vi "zahvat_cont.vi"   [LabVIEW 2017]
uses:
  <vilib>/myRIO/Instrument Drivers/Onboard IO/DIO/typedefs/DIO Reference.ctl
  <vilib>/myRIO/Common/Instrument Driver Framework/Utilities/typedefs/myRIO Generic Hardware Reference.ctl
  <vilib>/myRIO/Common/Instrument Driver Framework/Utilities/typedefs/Hardware Version Enum.ctl
  <vilib>/myRIO/Common/Instrument Driver Framework/Utilities/typedefs/myRIO v1.0 Reference.ctl
  <vilib>/myRIO/Common/Instrument Driver Framework/Utilities/typedefs/Generic FPGA Reference.ctl
  <vilib>/myRIO/Common/Instrument Driver Framework/myRIO v1.0/DIO/typedefs/DIO Channels List.ctl
  <vilib>/myRIO/Common/Instrument Driver Framework/myRIO v1.0/DIO/typedefs/DIO Channels Enum.ctl
  <vilib>/userdefined/High Color/nirio_resource_hc.ctl
  <vilib>/myRIO/Instrument Drivers/Onboard IO/PWM/typedefs/PWM Reference.ctl
  <vilib>/myRIO/Common/Instrument Driver Framework/myRIO v1.0/PWM/typedefs/PWM Channels Enum.ctl
  <vilib>/myRIO/Instrument Drivers/Onboard IO/PWM/typedefs/PWM Configuration.ctl
  <vilib>/myRIO/Common/Instrument Driver Framework/Utilities/vis/Is FPGA Ref Available.vi
  <vilib>/myRIO/Common/Instrument Driver Framework/myRIO v1.0/DIO/vis/myRIO v1.1 Open DIO.vi
  <vilib>/myRIO/Instrument Drivers/Onboard IO/DIO/vis/Write.vi
  <vilib>/myRIO/Common/Instrument Driver Framework/myRIO v1.0/PWM/vis/myRIO v1.1 Open PWM.vi
  <vilib>/myRIO/Instrument Drivers/Onboard IO/PWM/vis/Set Duty Cycle and Frequency.vi
  <vilib>/myRIO/Common/Instrument Driver Framework/Utilities/vis/Validate Channels.vi
  <vilib>/myRIO/Common/Instrument Driver Framework/myRIO v1.0/DIO/vis/myRIO v1.0 Reserve DIO.vi
  <vilib>/myRIO/Common/Instrument Driver Framework/myRIO v1.0/PWM/vis/myRIO v1.0 Reserve PWM.vi
  <vilib>/myRIO/Common/Instrument Driver Framework/myRIO v1.0/Resource Manager/vis/myRIO v1.0 Reserve Channel List.vi
  <vilib>/myRIO/Common/Instrument Driver Framework/myRIO v1.0/DIO/vis/myRIO v1.0 Build MUX Configuration DIO.vi
  <vilib>/myRIO/Common/Instrument Driver Framework/myRIO v1.0/PWM/vis/myRIO v1.0 Build MUX Configuration PWM.vi
  <vilib>/myRIO/Common/Instrument Driver Framework/myRIO v1.0/Resource Manager/vis/myRIO v1.0 Reserve Channel.vi
  <vilib>/myRIO/Common/Instrument Driver Framework/myRIO v1.0/Resource Manager/vis/myRIO v1.0 Unreserve Channel.vi
  <vilib>/myRIO/Common/Instrument Driver Framework/myRIO v1.0/Resource Manager/vis/myRIO v1.0 Create Configuration List.vi
  <vilib>/myRIO/Common/Instrument Driver Framework/myRIO v1.0/Resource Manager/vis/myRIO v1.0 Build Mutex Name.vi
  <vilib>/Utility/VariantDataType/GetNumericInfo.vi
  <vilib>/Utility/error.llb/Error Cluster From Error Code.vi
  <vilib>/myRIO/Common/Instrument Driver Framework/myRIO v1.0/myRIO v1.1 Open.vi
  <vilib>/myRIO/Common/Instrument Driver Framework/Utilities/vis/IO Manager.vi
  <vilib>/myRIO/Common/Instrument Driver Framework/Utilities/vis/Configuration Manager.vi
  <vilib>/myRIO/Common/Instrument Driver Framework/myRIO v1.0/Resource Manager/vis/myRIO v1.0 Configure IO.vi
  <vilib>/myRIO/Common/Instrument Driver Framework/myRIO v1.0/myRIO v1.0 Close.vi
  <vilib>/myRIO/Common/Instrument Driver Framework/myRIO v1.0/DIO/vis/myRIO v1.0 Write DIO.vi
  <vilib>/myRIO/Common/Instrument Driver Framework/myRIO v1.0/PWM/vis/myRIO v1.0 Write PWM.vi
  <vilib>/myRIO/Express VI/Onboard Devices/LED/LED Express VI.xnode
  <vilib>/myRIO/Instrument Drivers/Onboard IO/DIO/vis/myRIO DIO Open.xnode
  <vilib>/myRIO/Express VI/Onboard IO/PWM/PWM Express VI.xnode
  <vilib>/myRIO/Instrument Drivers/Onboard IO/PWM/vis/myRIO PWM Open.xnode
  <vilib>/myRIO/Instrument Drivers/Onboard IO/PWM/PWM.lvlib
  <vilib>/myRIO/Instrument Drivers/Onboard IO/DIO/DIO.lvlib
types:
  T1 = typedef "DIO.lvlib/DIO Reference.ctl" = cluster{"myRIO Reference":T2, "DIO Channels List":T6}
  T2 = typedef "myRIO Generic Hardware Reference.ctl" = cluster{"myRIO Model":T3, "myRIO Hardware Reference":T4}
  T3 = typedef "Hardware Version Enum.ctl" = enum16{"Unknown", "myRIO-1900", "myRIO-1950", "roboRIO", "NI ELVIS RIO CM"}
  T4 = typedef "myRIO v1.0 Reference.ctl" = cluster{"Generic FPGA Reference":T5, "Allow multiple opens":bool}
  T5 = typedef "Generic FPGA Reference.ctl" = refnum<k20>
  T6 = typedef "DIO Channels List.ctl" = T7[]
  T7 = typedef "DIO Channels Enum.ctl" = enum16{"Not Connected", "C/DIO0", "C/DIO1", "C/DIO2", "C/DIO3", "C/DIO4", "C/DIO5", "C/DIO6", "C/DIO7", "A/DIO0", "A/DIO1", "A/DIO2", "A/DIO3", "A/DIO4", "A/DIO5", "A/DIO6", "A/DIO7", "A/DIO8", "A/DIO9", "A/DIO10", "A/DIO11", "A/DIO12", "A/DIO13", "A/DIO14", "A/DIO15", "B/DIO0", "B/DIO1", "B/DIO2", "B/DIO3", "B/DIO4", "B/DIO5", "B/DIO6", "B/DIO7", "B/DIO8", "B/DIO9", "B/DIO10", "B/DIO11", "B/DIO12", "B/DIO13", "B/DIO14", "B/DIO15", "LED0", "LED1", "LED2", "LED3", "Button0", "DIO/DIO0", "DIO/DIO1", "DIO/DIO2", "DIO/DIO3", "DIO/DIO4", "DIO/DIO5", "DIO/DIO6", "DIO/DIO7", "DIO/DIO8", "DIO/DIO9", "SPI/CS0", "SPI/CS1", "SPI/CS2", "SPI/CS3", "LED RADIO (Green)", "LED RADIO (Red)", "LED COMM (Green)", "LED COMM (Red)", "LED MODE (Green)", "LED MODE (Red)"}
  T8 = typedef "nirio_resource_hc.ctl" = tag
  T9 = typedef "PWM.lvlib/PWM Reference.ctl" = cluster{"myRIO Reference":T2, "PWM Channels Enum":T10, "PWM Configuration":T11}
  T10 = typedef "PWM Channels Enum.ctl" = enum16{"Not Connected", "C/PWM0", "C/PWM1", "A/PWM0", "A/PWM1", "A/PWM2", "B/PWM0", "B/PWM1", "B/PWM2", "PWM/PWM0", "PWM/PWM1", "PWM/PWM2", "PWM/PWM3", "PWM/PWM4", "PWM/PWM5", "PWM/PWM6", "PWM/PWM7", "PWM/PWM8", "PWM/PWM9"}
  T11 = typedef "PWM.lvlib/PWM Configuration.ctl" = cluster{"Frequency":dbl, "Duty Cycle":dbl}
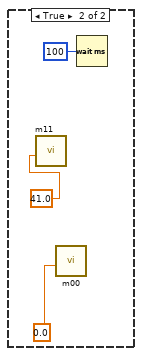
[diagram p3: hidden frame]
diagram:
  n1 = flat-sequence {
    frame #0 {
      n2 = Wait (ms)(milliseconds to wait=u32 1000) -> ()  [unwired: 1 out]
    }
    frame #1 {
      n3 = while {
        stop <- w3 stop-if-true
        n4 = call "ir2.vi"("Koffset [cm]"=0.0, "Kscale [cm-V]"=27.5) -> ("см"=w5:dbl)  [unwired: 8 in, 1 out]
        n5 = Less Or Equal?(x=w5, y=40.0) -> (x <= y?=w2:bool)
        n6 = case shown="True" w2 {
          frame False {
          }
          frame True {
            n7 = Wait (ms)(milliseconds to wait=u32 3000) -> ()  [unwired: 1 out]
          }
        }
        n8 = Not(x=w2) -> (.not. x?=w3:bool)
      }
    }
    frame #2 {
      n9 = flat-sequence {
        frame #0 {
          n10 = call "m11.vi"("position"=49.0) -> ()  [unwired: 10 in, 1 out]
          n11 = call "m00.vi"("position"=38.0) -> ()  [unwired: 10 in, 1 out]
          n12 = Wait (ms)(milliseconds to wait=u32 1650) -> ()  [unwired: 1 out]
        }
        frame #1 {
          n13 = call "m11.vi"("position"=0.0) -> ()  [unwired: 10 in, 1 out]
          n14 = call "m00.vi"("position"=0.0) -> ()  [unwired: 10 in, 1 out]
          n15 = Wait (ms)(milliseconds to wait=u32 1000) -> ()  [unwired: 1 out]
        }
        frame #2 {
          n16 = call "m00.vi"("position"=40.0) -> ()  [unwired: 10 in, 1 out]
          n17 = call "m11.vi"("position"=48.0) -> ()  [unwired: 10 in, 1 out]
          n18 = Wait (ms)(milliseconds to wait=u32 2950) -> ()  [unwired: 1 out]
        }
        frame #3 {
          w18 = TRUE ("LED0")
          n19 = call "m11.vi"("position"=0.0) -> ()  [unwired: 10 in, 1 out]
          n20 = xnode "LED"("LED0"=w18, "LED1"=w18, "LED2"=w18, "LED3"=w18) -> ()  [unwired: 1 in, 1 out]
          n21 = call "m00.vi"("position"=0.0) -> ()  [unwired: 10 in, 1 out]
          n22 = Wait (ms)(milliseconds to wait=u32 10000) -> ()  [unwired: 1 out]
        }
        frame #4 {
          w60 = FALSE ("LED0")
          n23 = xnode "LED 2"("LED0"=w60, "LED1"=w60, "LED2"=w60, "LED3"=w60) -> ()  [unwired: 1 in, 1 out]
        }
        frame #5 {
          n24 = call "line_sensor.vi"() -> ("line_true"=w99:bool)  [unwired: 10 in, 1 out]
          n25 = case shown="False" w99 {
            frame False {
              n26 = call "m11.vi"("position"=0.0) -> ()  [unwired: 10 in, 1 out]
              n27 = call "m00.vi"("position"=41.0) -> ()  [unwired: 10 in, 1 out]
              n28 = Wait (ms)(milliseconds to wait=u32 100) -> ()  [unwired: 1 out]
            }
            frame True {
              n29 = call "m11.vi"("position"=41.0) -> ()  [unwired: 10 in, 1 out]
              n30 = call "m00.vi"("position"=0.0) -> ()  [unwired: 10 in, 1 out]
              n31 = Wait (ms)(milliseconds to wait=u32 100) -> ()  [unwired: 1 out]
            }
          }
        }
        frame #6 {
          n32 = call "m11.vi"("position"=0.0) -> ()  [unwired: 10 in, 1 out]
          n33 = call "m00.vi"("position"=0.0) -> ()  [unwired: 10 in, 1 out]
        }
        frame #7 {
        }
        frame #8 {
          n34 = call "m11.vi"("position"=0.0) -> ()  [unwired: 10 in, 1 out]
          n35 = call "m00.vi"("position"=0.0) -> ()  [unwired: 10 in, 1 out]
          n36 = Wait (ms)(milliseconds to wait=u32 1000) -> ()  [unwired: 1 out]
        }
        frame #9 {
        }
      }
    }
    frame #3 {
      n37 = Wait (ms)(milliseconds to wait=u32 1000) -> ()  [unwired: 1 out]
    }
    frame #4 {
      n38 = while {
        stop <- w112 stop-if-true
        # "2,3"
        n39 = flat-sequence {
          tunnel: [w120] -> w117
          tunnel: [w133] -> w118
          tunnel: [w140] -> w116
          tunnel: [w146] -> w113
          frame #0 {
            n40 = while {
              tunnel: [w124] -> w120
              stop <- w126 stop-if-true
              # "37,5"
              # "37"
              n41 = call "m00.vi"("position"=40.0) -> ()  [unwired: 10 in, 1 out]
              n42 = call "m11.vi"("position"=0.0) -> ()  [unwired: 10 in, 1 out]
              n43 = call "line_sensor.vi"() -> ("line_true"=w126:bool)  [unwired: 10 in, 1 out]
              n44 = call "ir.vi"("Koffset [cm]"=0.0, "Kscale [cm-V]"=27.5) -> ("см"=w125:dbl)  [unwired: 8 in, 1 out]
              n45 = Less Or Equal?(x=w125, y=15.0) -> (x <= y?=w124:bool)
            }
            n46 = Wait (ms)(milliseconds to wait=u32 10) -> ()  [unwired: 1 out]
          }
          frame #1 {
            n47 = Wait (ms)(milliseconds to wait=u32 10) -> ()  [unwired: 1 out]
            n48 = call "m00.vi"("position"=0.0) -> ()  [unwired: 10 in, 1 out]
            n49 = call "ir.vi"("Koffset [cm]"=0.0, "Kscale [cm-V]"=27.5) -> ("см"=w134:dbl)  [unwired: 8 in, 1 out]
            n50 = call "m11.vi"("position"=0.0) -> ()  [unwired: 10 in, 1 out]
            n51 = Less Or Equal?(x=w134, y=15.0) -> (x <= y?=w133:bool)
          }
          frame #2 {
            # "37,5"
            # "41"
            n52 = call "m00.vi"("position"=0.0) -> ()  [unwired: 10 in, 1 out]
            n53 = call "m11.vi"("position"=41.0) -> ()  [unwired: 10 in, 1 out]
            n54 = call "ir.vi"("Koffset [cm]"=0.0, "Kscale [cm-V]"=27.5) -> ("см"=w141:dbl)  [unwired: 8 in, 1 out]
            n55 = Less Or Equal?(x=w141, y=15.0) -> (x <= y?=w140:bool)
            n56 = Wait (ms)(milliseconds to wait=u32 30) -> ()  [unwired: 1 out]
          }
          frame #3 {
            n57 = call "ir.vi"("Koffset [cm]"=0.0, "Kscale [cm-V]"=27.5) -> ("см"=w150:dbl)  [unwired: 8 in, 1 out]
            n58 = Less Or Equal?(x=w150, y=15.0) -> (x <= y?=w146:bool)
            n59 = call "m00.vi"("position"=0.0) -> ()  [unwired: 10 in, 1 out]
            n60 = call "m11.vi"("position"=0.0) -> ()  [unwired: 10 in, 1 out]
            n61 = Wait (ms)(milliseconds to wait=u32 10) -> ()  [unwired: 1 out]
          }
        }
        n62 = Or(x=w118, y=w117) -> (x .or. y?=w115:bool)
        n63 = Or(x=w116, y=w115) -> (x .or. y?=w114:bool)
        n64 = Or(x=w113, y=w114) -> (x .or. y?=w112:bool)
      }
    }
    frame #5 {
      n65 = call "m00.vi"("position"=0.0) -> ()  [unwired: 10 in, 1 out]
      n66 = call "m11.vi"("position"=0.0) -> ()  [unwired: 10 in, 1 out]
      n67 = Wait (ms)(milliseconds to wait=u32 1000) -> ()  [unwired: 1 out]
      n68 = Wait (ms)(milliseconds to wait=u32 100) -> ()  [unwired: 1 out]
    }
    frame #6 {
      w168 = 50.0 ("Frequency [Hz]")
      n69 = Divide(x=50.0, y=200.0) -> (x/y=w171:dbl)
      n70 = Add(x=w171, y=1.5) -> (x+y=w170:dbl)
      n71 = Divide(x=w170, y=1000.0) -> (x/y=w169:dbl)
      n72 = Multiply(x=w169, y=w168) -> (x*y=w172:dbl)
      n73 = call "M0.vi"("Duty Cycle"=0.5, "назад"=FALSE ("вперед"), "вперед"=FALSE ("назад")) -> ()  [unwired: 8 in, 1 out]
      n74 = call "M1.vi"("Duty Cycle"=0.5, "назад"=FALSE ("вперед"), "вперед"=FALSE ("назад")) -> ()  [unwired: 8 in, 1 out]
      n75 = xnode "PWM 8"("Duty Cycle"=w172, "Frequency [Hz]"=w168) -> ()  [unwired: 1 in, 1 out]
      n76 = Wait (ms)(milliseconds to wait=u32 1000) -> ()  [unwired: 1 out]
    }
    frame #7 {
      w212 = 50.0 ("Frequency [Hz]")
      w222 = 50.0 ("Frequency [Hz]")
      n77 = Divide(x=-40.0, y=200.0) -> (x/y=w225:dbl)
      n78 = Divide(x=-25.0, y=200.0) -> (x/y=w215:dbl)
      n79 = Add(x=w225, y=1.5) -> (x+y=w224:dbl)
      n80 = Add(x=w215, y=1.5) -> (x+y=w214:dbl)
      n81 = Divide(x=w224, y=1000.0) -> (x/y=w223:dbl)
      n82 = Divide(x=w214, y=1000.0) -> (x/y=w213:dbl)
      n83 = Multiply(x=w223, y=w222) -> (x*y=w226:dbl)
      n84 = Multiply(x=w213, y=w212) -> (x*y=w216:dbl)
      n85 = xnode "PWM"("Duty Cycle"=w226, "Frequency [Hz]"=w222) -> ()  [unwired: 1 in, 1 out]
      n86 = xnode "PWM 2"("Duty Cycle"=w216, "Frequency [Hz]"=w212) -> ()  [unwired: 1 in, 1 out]
      n87 = Wait (ms)(milliseconds to wait=u32 5000) -> ()  [unwired: 1 out]
    }
    frame #8 {
      w301 = 50.0 ("Frequency [Hz]")
      n88 = Divide(x=0.0, y=200.0) -> (x/y=w304:dbl)
      n89 = Add(x=w304, y=1.5) -> (x+y=w303:dbl)
      n90 = Divide(x=w303, y=1000.0) -> (x/y=w302:dbl)
      n91 = Multiply(x=w302, y=w301) -> (x*y=w305:dbl)
      n92 = xnode "PWM 4"("Duty Cycle"=w305, "Frequency [Hz]"=w301) -> ()  [unwired: 1 in, 1 out]
    }
    frame #9 {
      w346 = 50.0 ("Frequency [Hz]")
      n93 = Divide(x=200.0, y=200.0) -> (x/y=w349:dbl)
      n94 = Add(x=w349, y=1.5) -> (x+y=w348:dbl)
      n95 = Divide(x=w348, y=1000.0) -> (x/y=w347:dbl)
      n96 = Multiply(x=w347, y=w346) -> (x*y=w350:dbl)
      n97 = xnode "PWM 5"("Duty Cycle"=w350, "Frequency [Hz]"=w346) -> ()  [unwired: 1 in, 1 out]
      n98 = Wait (ms)(milliseconds to wait=u32 2000) -> ()  [unwired: 1 out]
    }
    frame #10 {
      w391 = 50.0 ("Frequency [Hz]")
      n99 = Divide(x=200.0, y=200.0) -> (x/y=w394:dbl)
      n100 = Add(x=w394, y=1.5) -> (x+y=w393:dbl)
      n101 = Divide(x=w393, y=1000.0) -> (x/y=w392:dbl)
      n102 = Multiply(x=w392, y=w391) -> (x*y=w395:dbl)
      n103 = xnode "PWM 6"("Duty Cycle"=w395, "Frequency [Hz]"=w391) -> ()  [unwired: 1 in, 1 out]
      n104 = Wait (ms)(milliseconds to wait=u32 25000) -> ()  [unwired: 1 out]
    }
    frame #11 {
      w436 = 50.0 ("Frequency [Hz]")
      n105 = Divide(x=0.0, y=200.0) -> (x/y=w439:dbl)
      n106 = Add(x=w439, y=1.5) -> (x+y=w438:dbl)
      n107 = Divide(x=w438, y=1000.0) -> (x/y=w437:dbl)
      n108 = Multiply(x=w437, y=w436) -> (x*y=w440:dbl)
      n109 = xnode "PWM 7"("Duty Cycle"=w440, "Frequency [Hz]"=w436) -> ()  [unwired: 1 in, 1 out]
      n110 = Wait (ms)(milliseconds to wait=u32 2000) -> ()  [unwired: 1 out]
    }
    frame #12 {
      n111 = call "m11.vi"("position"=40.0) -> ()  [unwired: 10 in, 1 out]
      n112 = call "m00.vi"("position"=38.0) -> ()  [unwired: 10 in, 1 out]
      n113 = Wait (ms)(milliseconds to wait=u32 1500) -> ()  [unwired: 1 out]
    }
    frame #13 {
      n114 = call "m11.vi"("position"=0.0) -> ()  [unwired: 10 in, 1 out]
      n115 = call "m00.vi"("position"=0.0) -> ()  [unwired: 10 in, 1 out]
    }
  }
